vi "DistPointLine.vi"(8 "P2":dbl[](array[numeric]), 9 "P1":dbl[](array[numeric]), 11 "Q":dbl[](array[numeric])) -> (2 "distance":dbl)   [LabVIEW 2017]
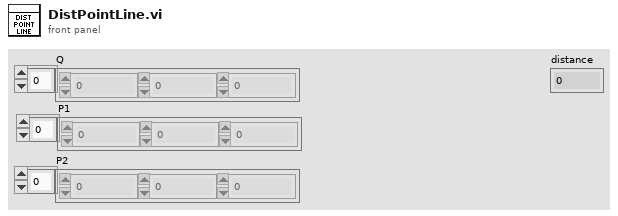
[diagram p1: front panel]
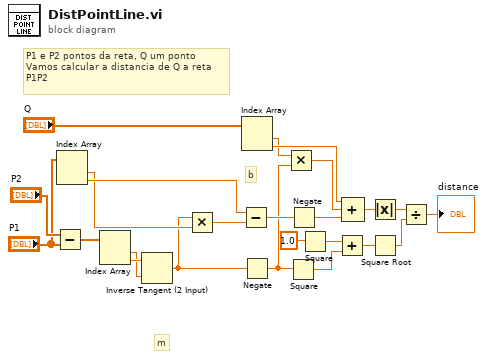
[diagram p0: block diagram]
diagram:
  # "b"
  # "m"
  # "P1 e P2 pontos da reta, Q um ponto\nVamos calcular a distancia de Q a reta \nP1P2"
  n1 = Subtract(x="P2", y="P1") -> (x-y=w23:dbl[])
  n2 = Index Array(array="P1") -> (element #1=w18:dbl, element #2=w19:dbl)  [unwired: 2 in]
  n3 = Index Array(array=w23) -> (element #1=w21:dbl, element #2=w22:dbl)  [unwired: 2 in]
  n4 = Inverse Tangent (2 Input)(1:w21, 2:w22) -> (0:w14:dbl)
  n5 = Multiply(x=w14, y=w18) -> (x*y=w17:dbl)
  n6 = Subtract(x=w19, y=w17) -> (x-y=w11:dbl)
  n7 = Index Array(array="Q") -> (element #1=w13:dbl, element #2=w15:dbl)  [unwired: 2 in]
  n8 = Negate(x=w14) -> (-x=w7:dbl)
  n9 = Multiply(x=w13, y=w7) -> (x*y=w12:dbl)
  n10 = Square(x=w7) -> (x^2=w5:dbl)
  n11 = Negate(x=w11) -> (-x=w10:dbl)
  n12 = Square(x=1.0) -> (x^2=w6:dbl)
  n13 = Add(x=w6, y=w5) -> (x+y=w4:dbl)
  n14 = Compound Arithmetic op=ADD(w15, w12, w10) -> (w9:dbl)
  n15 = Absolute Value(x=w9) -> (abs(x)=w3:dbl)
  n16 = Square Root(x=w4) -> (sqrt(x)=w2:dbl)
  n17 = Divide(x=w3, y=w2) -> (x/y=→"distance":dbl)
